vi "Matrix_ExtractColumnVector.vi"(10 "Column":i32, 11 "input matrix":T1) -> (0 "Error":bool, 3 "output column":T1)   [LabVIEW 2019, in "Trajectory_Library.lvlib"]
doc: "Creates a new LINEAR SYSTEM data cluster with the specified values. \n\n\nInputs: \n - XXX -- XXX.\n\nOutputs:\n - XXX -- XXX."
uses:
  Trajectory_Library.lvlib
  <vilib>/Analysis/Matrix/Datatypes/RealMatrix.ctl
  <vilib>/Analysis/Matrix/NI_Matrix.lvlib
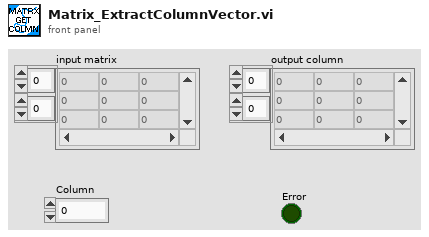
[diagram p1: front panel]
types:
  T1 = typedef "NI_Matrix.lvlib/RealMatrix.ctl" = dbl[][]
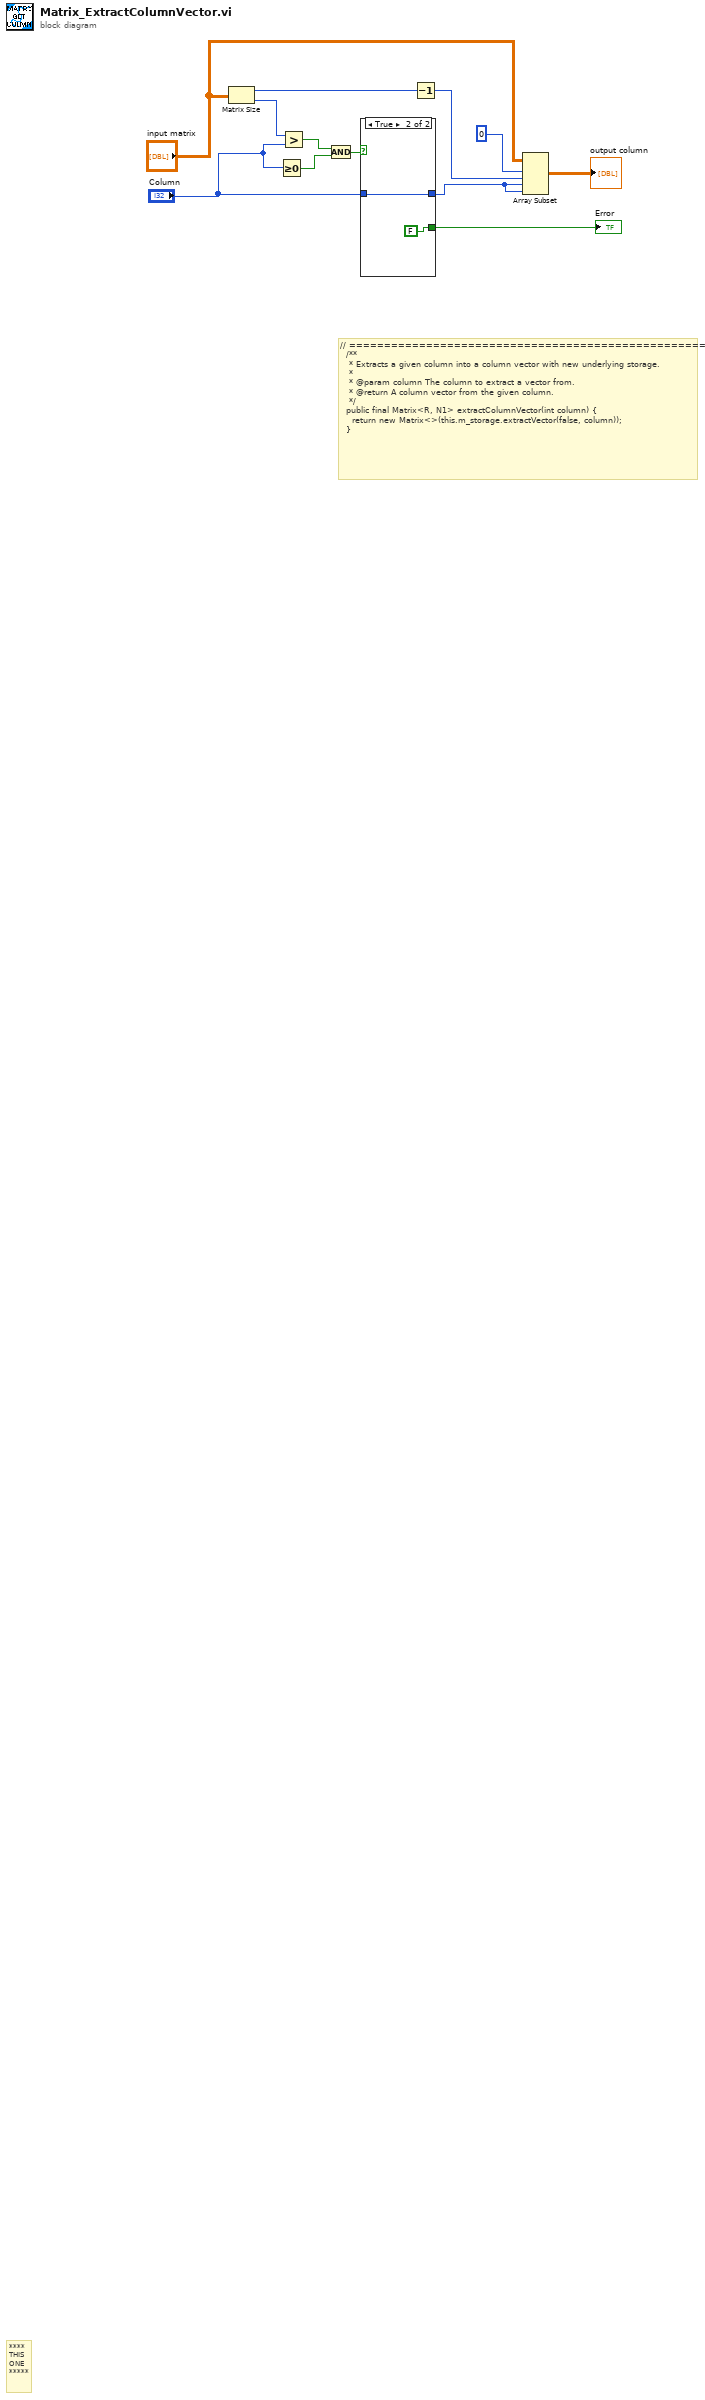
[diagram p0: block diagram]
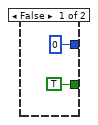
[diagram p2: hidden frame]
diagram:
  # "// ===================================================\n  /**\n   * Extracts a given column into a column vector with new underlying storage.\n   *\n   * @param column The column to extract a vector from.\n   * @return A column vector from the given column.\n   */\n  public final Matrix<R, N1> extractColumnVector(int column) {\n    return new Matrix<>(this.m_storage.extractVector(false, column));\n  }"
  # "****\nTHIS\nONE\n*****"
  n1 = Matrix Size(0:"input matrix") -> (1:w11:i32, 2:w7:i32)
  n2 = Greater Or Equal To 0?(x="Column") -> (x >= 0?=w8:bool)
  n3 = Greater?(x=w7, y="Column") -> (0:w9:bool)
  n4 = And(x=w9, y=w8) -> (x .and. y?=w1:bool)
  n5 = case shown="True" w1 {
    tunnel: "Column" -> [_ w16]
    tunnel: [0 ("Column") w16] -> w3
    tunnel: [TRUE FALSE] -> w2
    frame False {
    }
    frame True {
    }
  }
  "Error" <- w2
  n6 = Decrement(x=w11) -> (x-1=w5:i32)
  n7 = Array Subset(array="input matrix", index (row)=0 ("row 1"), length (row)=w5, index (col)=w3, length (col)=w3) -> (→"output column":T1)
